vi "Execute Line Test and Control.vi"(4 "Carpet Counter":dbl, 5 "Right Encoder RefNum":T1={"DevStatus"={"status"=FALSE, "code"=0, "source"=""}, "EncoderIndex"=enum."Invalid", "CounterIndex"=enum."Invalid", "DistancePerCount"=1.0, "Decoding Type"=enum."4x"}, 6 "Left Encoder RefNum":T1={"DevStatus"={"status"=FALSE, "code"=0, "source"=""}, "EncoderIndex"=enum."Invalid", "CounterIndex"=enum."Invalid", "DistancePerCount"=1.0, "Decoding Type"=enum."4x"}, 7 "Right":bool, 8 "Left":bool) -> (2 "Y-Axis To Drive":dbl, 3 "X-Axis To Drive":dbl)   [LabVIEW 2013]
uses:
  <vilib>/Rock Robotics/WPI/Encoder/WPI_EncoderDevRef.ctl
  <vilib>/Rock Robotics/SystemInterfaces/Encoder/FPGA_EncoderIdx.ctl
  <vilib>/Rock Robotics/SystemInterfaces/Counter/FPGA_CounterCtrSystemIndex.ctl
  <vilib>/Rock Robotics/WPI/Encoder/WPI_EncoderType.ctl
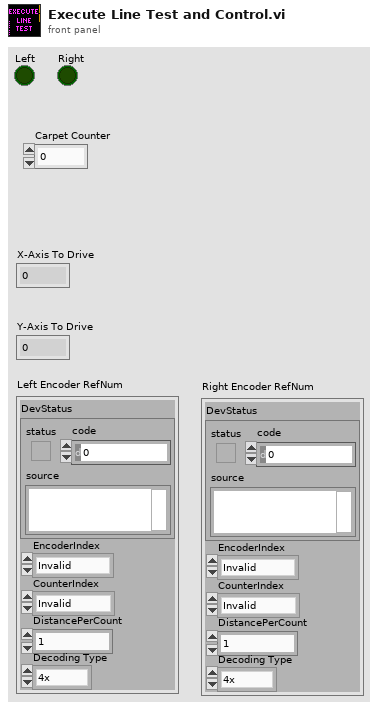
[diagram p1: front panel]
types:
  T1 = typedef "WPI_EncoderDevRef.ctl" = cluster{"DevStatus":errorcluster, "EncoderIndex":T2, "CounterIndex":T3, "DistancePerCount":dbl, "Decoding Type":T4}
  T2 = typedef "FPGA_EncoderIdx.ctl" = enum8{"Enc 0", "Enc 1", "Enc 2", "Enc 3", "Invalid"}
  T3 = typedef "FPGA_CounterCtrSystemIndex.ctl" = enum8{"Ctr 0", "Ctr 1", "Ctr 2", "Ctr 3", "Ctr 4", "Ctr 5", "Ctr 6", "Ctr 7", "Invalid"}
  T4 = typedef "WPI_EncoderType.ctl" = enum16{"1x", "2x", "4x"}
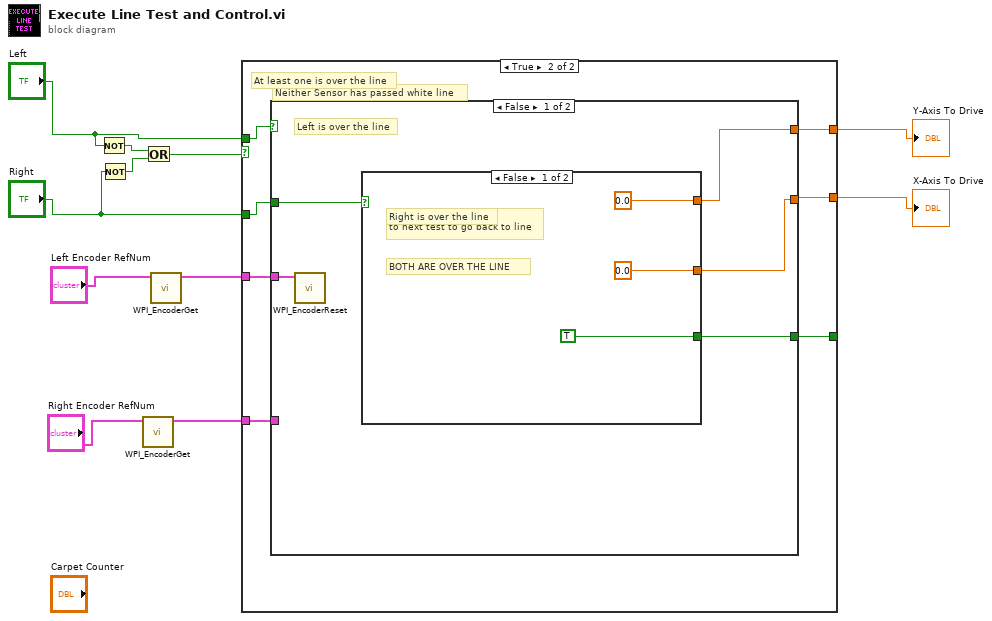
[diagram p0: block diagram]
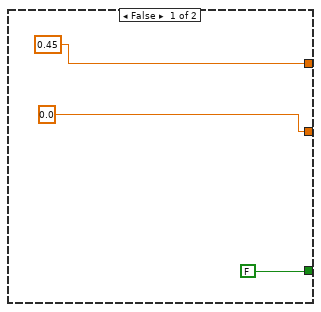
[diagram p2: hidden frame]
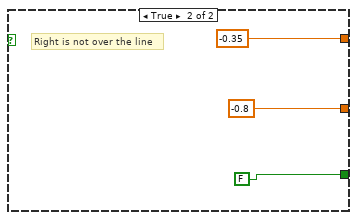
[diagram p3: hidden frame]
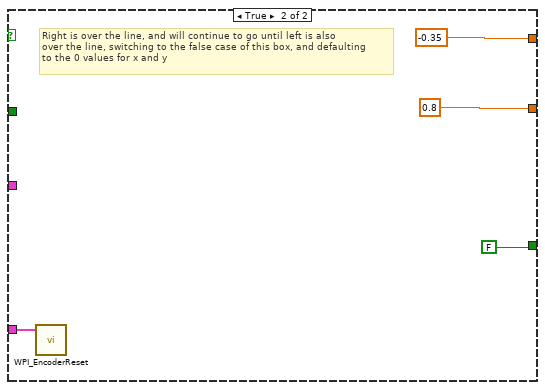
[diagram p4: hidden frame]
diagram:
  n1 = Not(x="Left") -> (.not. x?=w11:bool)
  n2 = Not(x="Right") -> (.not. x?=w10:bool)
  n3 = call <vilib>:"WPI_EncoderGet.vi"("EncoderDevRef"="Right Encoder RefNum") -> ("EncoderDevRef"=w3:T1)  [unwired: 5 in, 5 out]
  n4 = Or(x=w11, y=w10) -> (x .or. y?=w9:bool)
  n5 = call <vilib>:"WPI_EncoderGet.vi"("EncoderDevRef"="Left Encoder RefNum") -> ("EncoderDevRef"=w4:T1)  [unwired: 5 in, 5 out]
  n6 = case shown="True" w9 {
    tunnel: "Left" -> [_ w21]
    tunnel: "Right" -> [_ w20]
    tunnel: [0.45 ("Y-Axis To Drive") w19] -> w2
    tunnel: [0.0 ("X-Axis To Drive") w18] -> w1
    tunnel: w4 -> [_ w17]
    tunnel: w3 -> [_ w16]
    tunnel: [FALSE w15] -> _
    frame False {
    }
    frame True {
      # "At least one is over the line"
      # "Neither Sensor has passed white line"
      n7 = case shown="False" w21 {
        tunnel: [w24 0.8 ("X-Axis To Drive")] -> w18
        tunnel: [w25 -0.35 ("X-Axis To Drive")] -> w19
        tunnel: w20 -> [w26 _]
        tunnel: w17 -> [w23 _]
        tunnel: w16 -> [_ w34]
        tunnel: [w22 FALSE] -> w15
        frame False {
          # "Left is over the line"
          n8 = call <vilib>:"WPI_EncoderReset.vi"("EncoderDevRef"=w23) -> ()  [unwired: 9 in, 2 out]
          n9 = case shown="False" w26 {
            tunnel: [0.0 ("X-Axis To Drive") -0.35 ("X-Axis To Drive")] -> w25
            tunnel: [0.0 ("X-Axis To Drive") -0.8 ("X-Axis To Drive")] -> w24
            tunnel: [TRUE FALSE] -> w22
            frame False {
              # "true constant to send\nto next test to go back to line"
              # "BOTH ARE OVER THE LINE"
              # "Right is over the line"
            }
            frame True {
              # "Right is not over the line"
            }
          }
        }
        frame True {
          # "Right is over the line, and will continue to go until left is also\nover the line, switching to the false case of this box, and defaulting\nto the 0 values for x and y"
          n10 = call <vilib>:"WPI_EncoderReset.vi"("EncoderDevRef"=w34) -> ()  [unwired: 9 in, 2 out]
        }
      }
    }
  }
  "X-Axis To Drive" <- w1
  "Y-Axis To Drive" <- w2
